vi "ACIR.vi"() -> (2 "Voltage":dbl, 3 "AC IR (milliohm)":dbl)   [LabVIEW 2024]
uses:
  <vilib>/numeric/Random Number (Range) DBL.vi
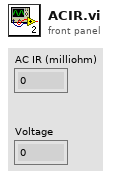
[diagram p1: front panel]
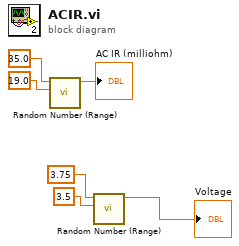
[diagram p0: block diagram]
diagram:
  n1 = call-poly <vilib>:"Random Number (Range).vi"("lower bound (0)"=19.0, "upper bound (100)"=35.0) -> ("number"=→"AC IR (milliohm)":dbl)  [unwired: 9 in]
  n2 = call-poly <vilib>:"Random Number (Range).vi"("lower bound (0)"=3.5, "upper bound (100)"=3.75) -> ("number"=→"Voltage":dbl)  [unwired: 9 in]
